vi "飞.vi"(8 "error in (no error)":errorcluster caption="错误输入（无错误）", 11 "绿头鸭 输入":refnum<class "绿头鸭.lvclass">) -> (0 "error out":errorcluster caption="错误输出", 3 "绿头鸭 输出":refnum<class "绿头鸭.lvclass">)   [LabVIEW 2022 SP3, in "鸭子库.lvlib" / "绿头鸭.lvclass"]
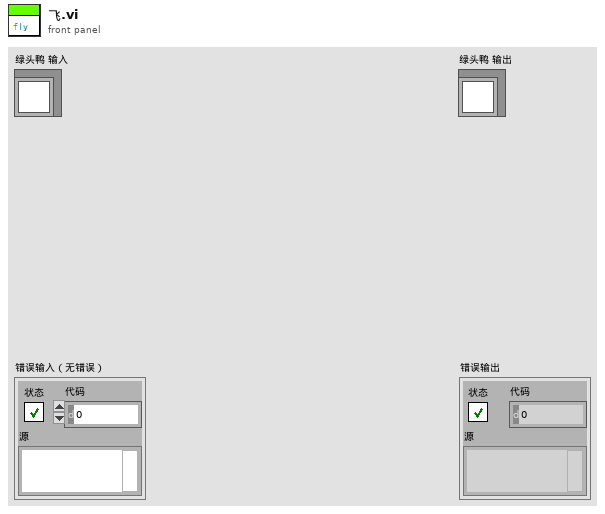
[diagram p1: front panel]
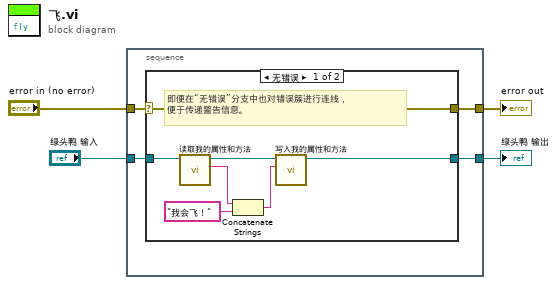
[diagram p0: block diagram]
diagram:
  n1 = stacked-sequence {
    tunnel: [w6] -> w4
    tunnel: [w8] -> w3
    tunnel: "error in (no error)" -> [w5]
    tunnel: "绿头鸭 输入" -> [w7]
    frame #0 {
      n2 = case shown="无错误" w5 {
        selector: w5 -> [w15 w17]
        tunnel: [w15 w17] -> w6
        tunnel: [w9 w16] -> w8
        tunnel: w7 -> [w10 w16]
        frame No Error {
          # "即便在“无错误”分支中也对错误簇进行连线，\n便于传递警告信息。"
          n3 = call "读取我的属性和方法.vi"("鸭子输入"=w10) -> ("我的属性和方法"=w14:string, "鸭子输出"=w11:refnum<class "绿头鸭.lvclass">)  [unwired: 8 in, 1 out]
          n4 = Concatenate Strings(w14, "我会飞！" ("字符串")) -> (w12:string)
          n5 = call "写入我的属性和方法.vi"("我的属性和方法"=w12, "鸭子输入"=w11) -> ("鸭子输出"=w9:refnum<class "绿头鸭.lvclass">)  [unwired: 8 in, 1 out]
        }
        frame Error {
        }
      }
    }
  }
  "error out" <- w4
  "绿头鸭 输出" <- w3
